vi "MGCC_FntStaMach_restart.vi"(6 "Timeout (180,000 ms)":u32=180000, 7 "Wait Until Complete (T)":bool=TRUE, 8 "error in (no error)":errorcluster, 9 "Flush DNS (F)":bool, 10 "Install Mode (F)":bool, 11 "Session in":refnum<k21>) -> (0 "error out":errorcluster, 2 "New IP Address":string, 3 "Session out":refnum<k21>)   [LabVIEW 2016]
doc: "-----------------------------------------------------------------------------------------------------------------------\nCopyright <2019> <The University of Tennessee at Knoxville and the University of Tennessee Research Foundation>\nThis software is released under BSD-3 \nhttps://opensource.org/licenses/BSD-3-Clause \nAdditional license options available at https://utrf.tennessee.edu/industry/sample-agreements/\n-----------------------------------------------------------------------------------------------------------------------\n\nReboots a system or network device."
uses:
  <vilib>/Utility/error.llb/Error Cluster From Error Code.vi
  <vilib>/nisyscfg/nisyscfg.lvlib
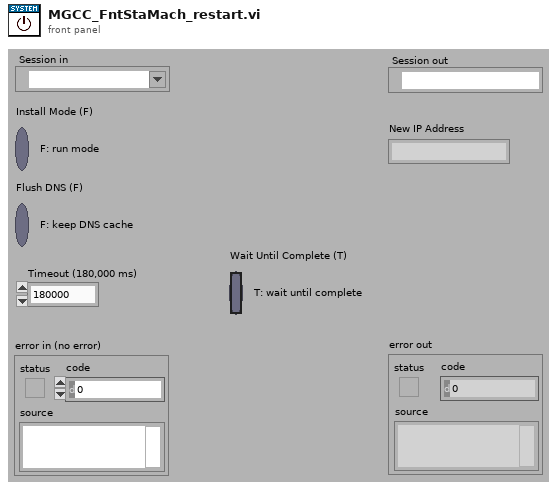
[diagram p1: front panel]
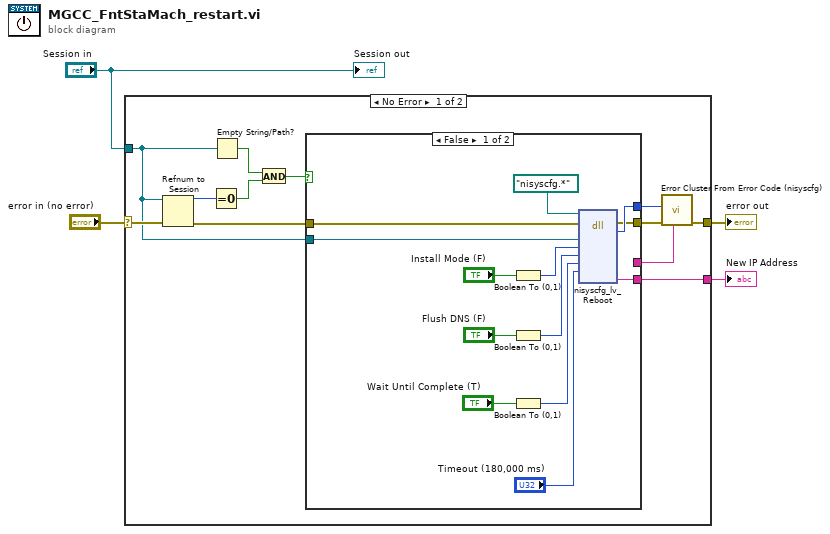
[diagram p0: block diagram]
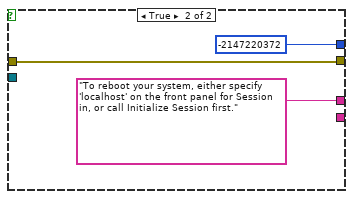
[diagram p2: hidden frame]
diagram:
  n1 = case shown="No Error" "error in (no error)" {
    selector: "error in (no error)" -> [w12 w33]
    tunnel: [w16 _] -> w4
    tunnel: [w13 w33] -> w3
    tunnel: "Session in" -> [w10 _]
    frame No Error {
      n2 = Refnum to Session(4:w12, 7:w10) -> (0:w11:errorcluster, 3:w9:u64)
      n3 = Equal To 0?(x=w9) -> (x = 0?=w7:bool)
      n4 = Empty String/Path?(string/path=w10) -> (empty?=w8:bool)
      n5 = And(x=w8, y=w7) -> (x .and. y?=w6:bool)
      n6 = case shown="False" w6 {
        tunnel: [w28 _] -> w16
        tunnel: [w27 -2147220372 ("result")] -> w15
        tunnel: [w26 w32] -> w14
        tunnel: w11 -> [w18 w32]
        tunnel: w10 -> [w17 _]
        tunnel: [_ "To reboot your system, either specify 'localhost' on the front panel for Session in, or call Initialize Session first."] -> w5
        frame False {
          n7 = Boolean To (0,1)(Boolean="Install Mode (F)") -> (0, 1=w22:i16)
          n8 = Boolean To (0,1)(Boolean="Flush DNS (F)") -> (0, 1=w21:i16)
          n9 = Boolean To (0,1)(Boolean="Wait Until Complete (T)") -> (0, 1=w20:i16)
          n10 = dll-call lib="nisyscfg.*" fn="nisyscfg_lv_Reboot" label="Reboot"(path in=path "nisyscfg.*", error in=w18, "system"=w17, "installMode"=w22, "flushDNS"=w21, "waitUntilComplete"=w20, "timeout"="Timeout (180,000 ms)") -> (error out=w26:errorcluster, "result"=w27:i32, "new IP"=w28:string)  [unwired: 7 in, 1 out]
        }
        frame True {
        }
      }
      n11 = call <vilib>:"Error Cluster From Error Code (nisyscfg).vi"("Details String"=w5, "error in (no error)"=w14, "Error Code (0)"=w15) -> ("error out"=w13:errorcluster)  [unwired: 8 in]
    }
    frame Error {
    }
  }
  "error out" <- w3
  "New IP Address" <- w4
  "Session out" <- "Session in"
